vi "test image processing.vi"() -> ()   [LabVIEW 2015]
uses:
  <vilib>/picture/picture.llb/Draw True-Color Pixmap.vi
panel:
  out "error out":errorcluster
  out "Reagent Pic 1":picture
  out "Downloaded Picture 7":picture
  out "Downloaded Picture 6":picture
  out "Downloaded Picture 5":picture
  out "Downloaded Picture 4":picture
  out "Downloaded Picture 3":picture
  out "Downloaded Picture 2":picture
  out "Downloaded Picture":picture
  in  "Product":string
  in  "Synthesis Route Array":string[][](array[string])=[["Benzaldehyde", "Benzylamine", "Acetic acid ", "Na(BH3)CN", "", ""]]
  # "+"
  # "+"
  # "+"
  # "+"
  # "+"
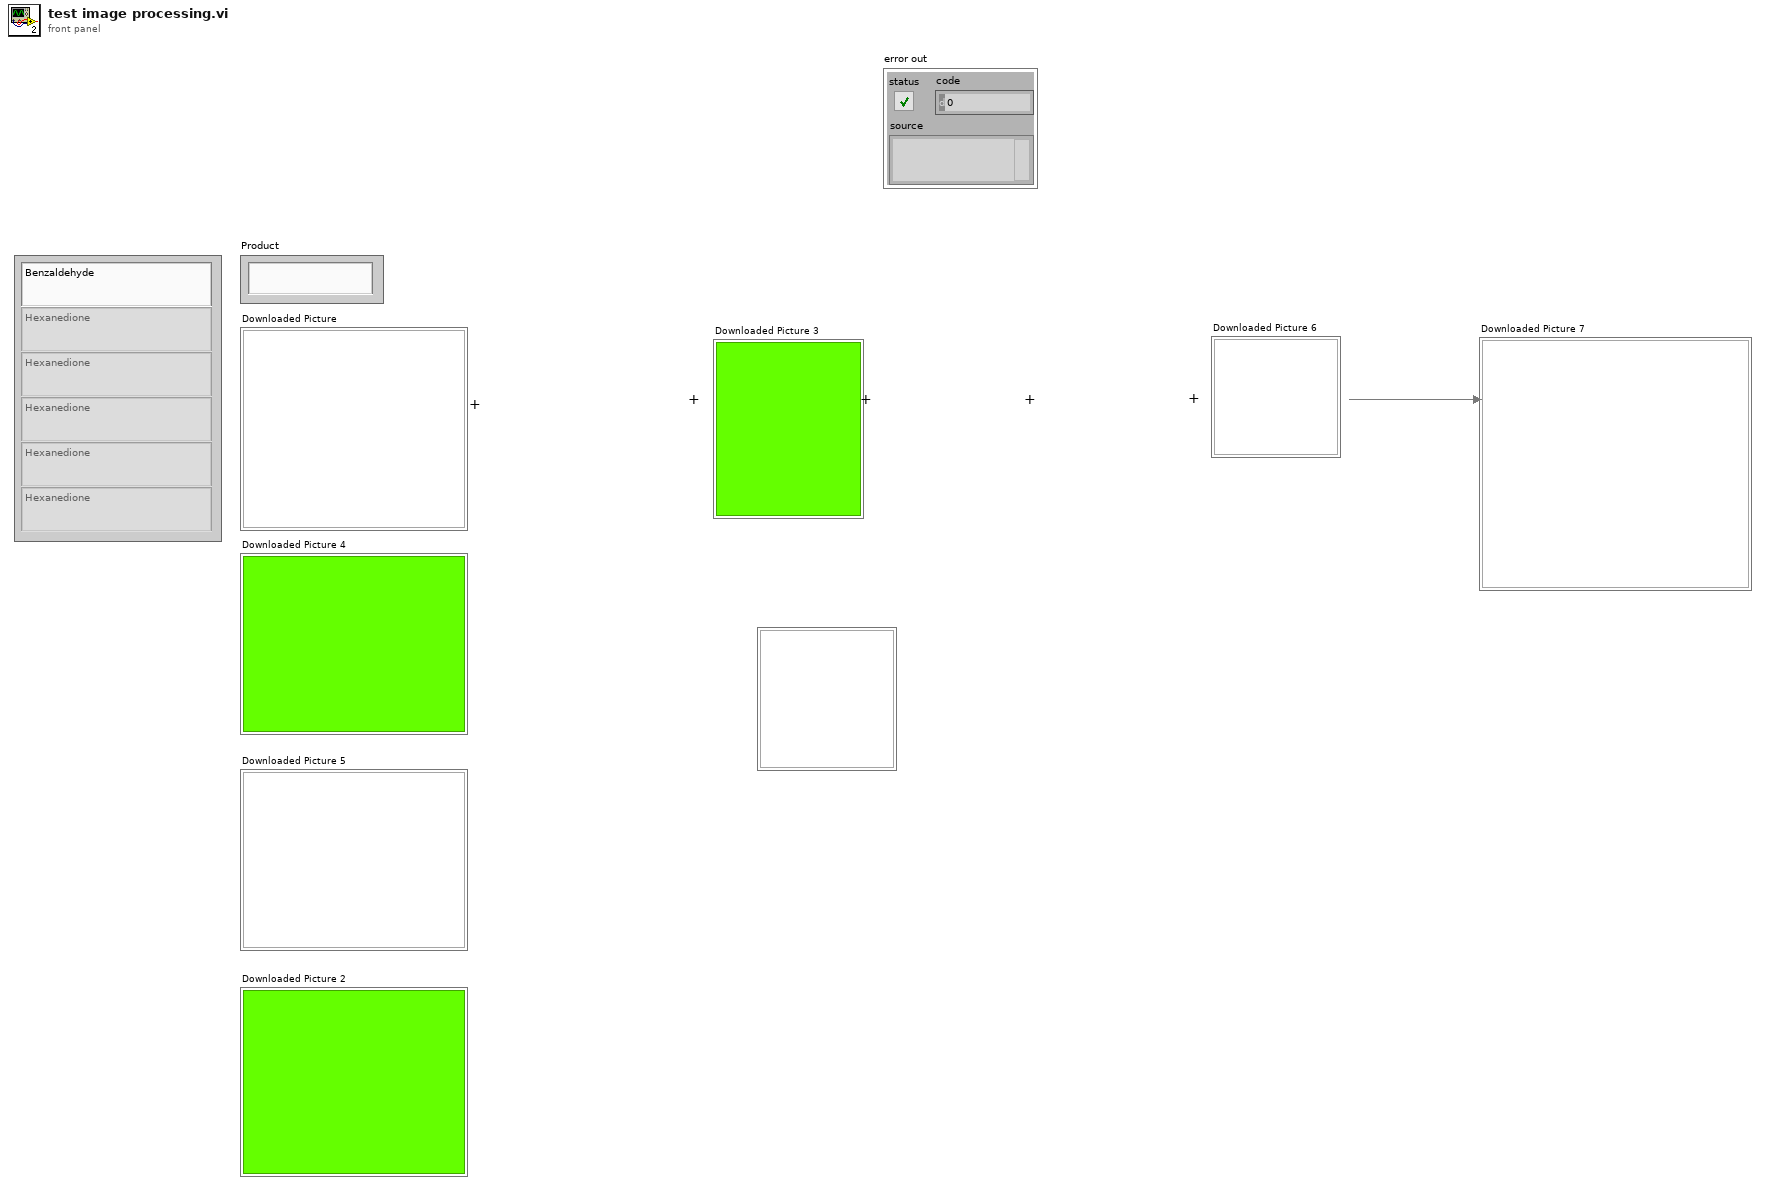
[diagram p1: front panel]
types:
  T1 = typedef "imagedata.ctl" = cluster{"image type":i32, "image depth":i32, "image":u8[], "mask":u8[], "colors":u32[], "Rectangle":cluster{"left":i16, "top":i16, "right":i16, "bottom":i16}}
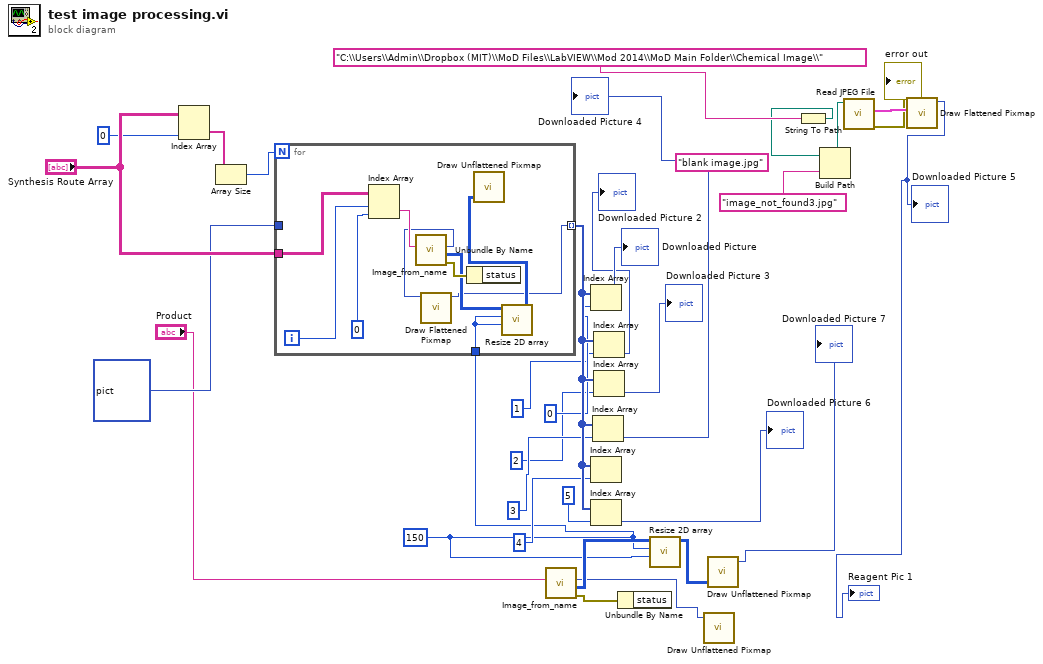
[diagram p0: block diagram]
diagram:
  (unwired) "blank image.jpg" ("name or relative path")
  w10 = 150 ("New Height")
  n1 = Index Array(array="Synthesis Route Array", index (col)=0 ("disabled index (col)")) -> (element=w28:string[])  [unwired: 1 in]
  n2 = Array Size(array=w28) -> (size(s)=w31:i32)
  n3 = for {
    N: w31 -> [_]
    tunnel: "Synthesis Route Array" -> [w41]
    tunnel: picture data[5B] ("Downloaded Picture") -> [_]
    tunnel: [w32] -> w26 mode=indexing
    tunnel: w10 -> [w34]
    i -> [w39]
    n4 = Index Array(array=w41, index (row)=w39, index (col)=0 ("disabled index (col)")) -> (element=w40:string)
    n5 = call "Image_from_name.vi"("Chemical Name"=w40) -> ("error out"=w37:errorcluster, "24-bit pixmap"=w36:u32[][], "Downloaded Picture"=w33:picture)  [unwired: 8 in]
    n6 = call <vilib>:"Draw Flattened Pixmap.vi"("picture"=w33) -> ("new picture"=w32:picture)  [unwired: 8 in]
    n7 = Unbundle By Name(w37) -> ()  [unwired: 1 out]
    n8 = call "Resize 2D array.vi"("New Width"=w34, "New Height"=w34, "2D Array In"=w36) -> ("Resized Array"=w35:u32[][])  [unwired: 4 in]
    n9 = call-poly <vilib>:"Draw Unflattened Pixmap.vi"("data (RGB format)"=w35) -> ()  [unwired: 8 in, 1 out]
  }
  n10 = call "Image_from_name.vi"("Chemical Name"="Product") -> ("error out"=w14:errorcluster, "24-bit pixmap"=w11:u32[][], "Downloaded Picture"=w4:picture)  [unwired: 8 in]
  n11 = Index Array(array=w26, index=0 ("disabled index (col)")) -> (element=→"Downloaded Picture":picture)
  n12 = Index Array(array=w26, index=4 ("disabled index (col)")) -> ()  [unwired: 1 out]
  n13 = Index Array(array=w26, index=5 ("disabled index (col)")) -> (element=→"Downloaded Picture 6":picture)
  n14 = Index Array(array=w26, index=3 ("disabled index (col)")) -> (element=→"Downloaded Picture 4":picture)
  n15 = Index Array(array=w26, index=1 ("disabled index (col)")) -> (element=→"Downloaded Picture 2":picture)
  n16 = Index Array(array=w26, index=2 ("disabled index (col)")) -> (element=→"Downloaded Picture 3":picture)
  n17 = Unbundle By Name(w14) -> ()  [unwired: 1 out]
  n18 = call "Resize 2D array.vi"("New Width"=w10, "New Height"=w10, "2D Array In"=w11) -> ("Resized Array"=w12:u32[][])  [unwired: 4 in]
  n19 = call-poly <vilib>:"Draw Unflattened Pixmap.vi"("picture"=w4) -> ()  [unwired: 8 in, 1 out]
  n20 = call-poly <vilib>:"Draw Unflattened Pixmap.vi"("data (RGB format)"=w12) -> ("new picture"=→"Downloaded Picture 7":picture)  [unwired: 8 in]
  n21 = String To Path(string="C:\\Users\\Admin\\Dropbox (MIT)\\MoD Files\\LabVIEW\\Mod 2014\\MoD Main Folder\\Chemical Image\\") -> (path=w7:path)
  n22 = Build Path(base path=w7, name or relative path="image_not_found3.jpg") -> (appended path=w6:path)
  n23 = call <vilib>:"Read JPEG File.vi"("path to JPEG file"=w6) -> ("error out"=→"error out":errorcluster, "image data"=w9:T1)  [unwired: 1 in, 8 out]
  n24 = call <vilib>:"Draw Flattened Pixmap.vi"("image data"=w9) -> ("new picture"=→"Downloaded Picture 5" →"Reagent Pic 1":picture)  [unwired: 3 in, 5 out]
